vi "1D Auto Correlation (DBL).vi"(10 "normalization":enum32{"none", "unbiased", "biased"}(ring), 11 "X":dbl[](array[numeric])) -> (0 "error":i32, 3 "Rxx":dbl[](array[numeric]))   [LabVIEW 2010, in "NI_AALPro.lvlib"]
doc: "Computes the autocorrelation of the input sequence <B>X</B>. Wire data to the <B>X</B> input to determine the polymorphic instance to use or manually select the instance."
uses:
  NI_AALPro.lvlib
  lvanlys.dll
panel:
  # "1D AutoCorrelation (DBL)"
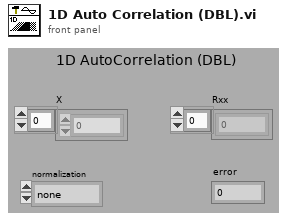
[diagram p1: front panel]
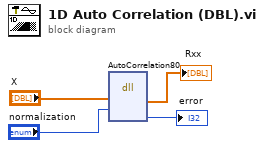
[diagram p0: block diagram]
diagram:
  n1 = dll-call lib="C:/Program Files/National Instruments/LabVIEW 2010/resource/lvanlys.*" fn="AutoCorrelation80"("X"="X", "norm"="normalization") -> ("X"=→"Rxx":dbl[], "error"=→"error":i32)  [unwired: 6 in, 2 out]
